vi "HFRR ADV v016 new software.vi"() -> ()   [LabVIEW 2025] (continued)
        n324 = event-data() -> ()  [unwired: 1 in, 6 out]
        n325 = Unbundle By Name("Password 3") -> ("Service Password"=w414:string)
        n326 = call <vilib>:"Trim Whitespace.vi"("string"=w414) -> ("trimmed string"=w412:string)  [unwired: 1 in]
        n327 = Equal?(x=w412, y="Service@123") -> (x = y?=w413:bool)
        n328 = case shown="False" w413 {
          selector: w413 -> [w418 w420]
          frame False {
            n329 = local write "Service Password enable"(w418) -> ()
            n330 = property on="Service Password Log" class="Str"("Visible"=TRUE) -> ()  [unwired: 2 in, 2 out]
            n331 = property on="Tab Control 5" class="TabCtl (strict)"("Tabs Visible?"=TRUE ("Page Labels Display Visible?")) -> ()  [unwired: 2 in, 2 out]
          }
          frame True {
            n332 = property on="Service Password Log" class="Str"("Visible"=FALSE) -> ()  [unwired: 2 in, 2 out]
            "Service Password enable" <- w420
          }
        }
      }
      event "Sign In": Value Change {
        w422 = FALSE ("Visible")
        n333 = event-data() -> ()  [unwired: 1 in, 6 out]
        n334 = property on="About" class="Clust (strict)"("Visible"=w422) -> ()  [unwired: 2 in, 2 out]
        n335 = property on="Password 3" class="Clust (strict)"("Visible"=w422) -> ()  [unwired: 2 in, 2 out]
        n336 = property on="Service Password Log" class="Str"("Visible"=FALSE) -> ()  [unwired: 2 in, 2 out]
      }
      event "Info": Value Change {
        n337 = event-data() -> ()  [unwired: 1 in, 6 out]
        n338 = local read "Info"() -> (w424:bool)
        n339 = case shown="False" w424 {
          frame False {
            n340 = property on="About" class="Clust (strict)"("Visible"=FALSE) -> ()  [unwired: 2 in, 2 out]
          }
          frame True {
            n341 = property on="About" class="Clust (strict)"("Visible"=TRUE) -> ()  [unwired: 2 in, 2 out]
          }
        }
      }
      event "Calibration": Value Change {
        n342 = event-data() -> ()  [unwired: 1 in, 6 out]
        n343 = local read "Calibration"() -> (w428:bool)
        n344 = case shown="False" w428 {
          frame False {
            n345 = property on="Calibration 2" class="TabCtl (strict)"("Visible"=FALSE) -> ()  [unwired: 2 in, 2 out]
            n346 = local write "Cal Password"("" ("Cal Password")) -> ()
          }
          frame True {
            n347 = property on="Calibration 2" class="TabCtl (strict)"("Visible"=TRUE) -> ()  [unwired: 2 in, 2 out]
            n348 = local write "Cal Password"("" ("Cal Password")) -> ()
          }
        }
        n349 = property on="Wrong Password" class="Str"("Visible"=FALSE) -> ()  [unwired: 2 in, 2 out]
      }
      event "Cal Password": Value Change {
        n350 = event-data() -> ()  [unwired: 1 in, 6 out]
        n351 = local read "Cal Password"() -> (w436:string)
        n352 = call <vilib>:"Trim Whitespace.vi"("string"=w436) -> ("trimmed string"=w435:string)  [unwired: 1 in]
        n353 = Equal?(x=w435, y="Cal@321") -> (x = y?=w433:bool)
        n354 = case shown="True" w433 {
          frame False {
            n355 = property on="Wrong Password" class="Str"("Visible"=TRUE) -> ()  [unwired: 2 in, 2 out]
          }
          frame True {
            n356 = property on="Wrong Password" class="Str"("Visible"=FALSE) -> ()  [unwired: 2 in, 2 out]
            n357 = local write "Main Tab"(T2."About" ("Main Tab")) -> ()
            n358 = local write "Cal Password"("" ("Cal Password")) -> ()
            n359 = local write "Main Dashboard Buttons"(T1."About" ("Main Dashboard Buttons")) -> ()
            n360 = local write "Tab Control 5"(T12."Temperature Calibration" ("Tab Control 5")) -> ()
            n361 = property on="Calibration 2" class="TabCtl (strict)"("Visible"=FALSE) -> ()  [unwired: 2 in, 2 out]
            n362 = property on="Tab Control 5" class="TabCtl (strict)"("Tabs Visible?"=FALSE ("Page Labels Display Visible?")) -> ()  [unwired: 2 in, 2 out]
            n363 = local write "Calibration"(FALSE ("Calibration")) -> ()
          }
        }
      }
      event "Calibration Selection": Value Change {
        n364 = event-data() -> ()  [unwired: 1 in, 6 out]
        n365 = local read "Calibration Selection"() -> (w447:T8)
        n366 = case shown="\"Stroke Calibration\"" w447 {
          tunnel: [T7."Stroke" ("Main Calibration Tab") T7."Friction" ("Main Calibration Tab") T7."Main" ("Main Calibration Tab") T7."Temperature" ("Main Calibration Tab")] -> w446
          frame "Stroke Calibration" {
          }
          frame "Friction Force Calibration" {
          }
          frame Default {
          }
          frame "Temperature Calibration" {
          }
        }
        n367 = local write "Main Calibration Tab"(w446) -> ()
      }
      event "Back Stroke": Value Change {
        n368 = event-data() -> ()  [unwired: 1 in, 6 out]
        n369 = local write "Main Stroke Tab"(T9."Step 1" ("Main Stroke Tab")) -> ()
        n370 = local write "Main Calibration Tab"(T7."Main" ("Main Calibration Tab")) -> ()
        n371 = local write "Back Stroke"(FALSE ("Back Stroke")) -> ()
      }
      event "Step 2 Back": Value Change {
        n372 = event-data() -> ()  [unwired: 1 in, 6 out]
        n373 = local write "Main Stroke Tab"(T9."Step 1" ("Main Stroke Tab")) -> ()
        n374 = local write "Step 2 Back"(FALSE ("Back Stroke")) -> ()
      }
      event "Step 3 Back": Value Change {
        n375 = event-data() -> ()  [unwired: 1 in, 6 out]
        n376 = local write "Main Stroke Tab"(T9."Step 2" ("Main Stroke Tab")) -> ()
        n377 = local write "Step 3 Back"(FALSE ("Back Stroke")) -> ()
      }
      event "Step 4 Back": Value Change {
        n378 = event-data() -> ()  [unwired: 1 in, 6 out]
        n379 = local write "Main Stroke Tab"(T9."Step 3" ("Main Stroke Tab")) -> ()
        n380 = local write "Step 4 Back"(FALSE ("Back Stroke")) -> ()
      }
      event "Step 5 Back": Value Change {
        n381 = event-data() -> ()  [unwired: 1 in, 6 out]
        n382 = local write "Main Stroke Tab"(T9."Step 4" ("Main Stroke Tab")) -> ()
        n383 = local write "Step 5 Back"(FALSE ("Back Stroke")) -> ()
      }
      event "Step 6 Back": Value Change {
        n384 = event-data() -> ()  [unwired: 1 in, 6 out]
        n385 = local write "Main Stroke Tab"(T9."Step 5" ("Main Stroke Tab")) -> ()
        n386 = local write "Step 6 Back"(FALSE ("Back Stroke")) -> ()
      }
      event "Back Stroke step 7": Value Change {
        n387 = event-data() -> ()  [unwired: 1 in, 6 out]
        n388 = local write "Main Stroke Tab"(T9."Step 6" ("Main Stroke Tab")) -> ()
        n389 = local write "Back Stroke step 7"(FALSE ("Back Stroke")) -> ()
      }
      event "Back Stroke step 8": Value Change {
        n390 = event-data() -> ()  [unwired: 1 in, 6 out]
        n391 = local write "Main Stroke Tab"(T9."Step 7" ("Main Stroke Tab")) -> ()
        n392 = local write "Back Stroke step 8"(FALSE ("Back Stroke")) -> ()
      }
      event "Back Stroke 8": Value Change {
        n393 = event-data() -> ()  [unwired: 1 in, 6 out]
        n394 = local write "MOVE CARRIAGE TO"(0.2 ("MOVE CARRIAGE TO")) -> ()
        n395 = local write "Main Stroke Tab"(T9."Step 1" ("Main Stroke Tab")) -> ()
        n396 = local write "Back Stroke 8"(FALSE ("Back Stroke 8")) -> ()
      }
      event "Continue Stroke": Value Change {
        n397 = event-data() -> ()  [unwired: 1 in, 6 out]
        n398 = local write "Main Stroke Tab"(T9."Step 2" ("Main Stroke Tab")) -> ()
        n399 = local write "Continue Stroke"(FALSE ("Continue Stroke")) -> ()
      }
      event "Continue Stroke step 2": Value Change {
        n400 = event-data() -> ()  [unwired: 1 in, 6 out]
        n401 = local write "Main Stroke Tab"(T9."Step 3" ("Main Stroke Tab")) -> ()
        n402 = local write "Continue Stroke step 2"(FALSE ("Continue Stroke")) -> ()
      }
      event "Continue Stroke step 3": Value Change {
        n403 = event-data() -> ()  [unwired: 1 in, 6 out]
        n404 = local write "Main Stroke Tab"(T9."Step 4" ("Main Stroke Tab")) -> ()
        n405 = local write "Continue Stroke step 3"(FALSE ("Continue Stroke")) -> ()
      }
      event "Continue Stroke step 4": Value Change {
        n406 = event-data() -> ()  [unwired: 1 in, 6 out]
        n407 = local write "Main Stroke Tab"(T9."Step 5" ("Main Stroke Tab")) -> ()
        n408 = local write "Continue Stroke step 4"(FALSE ("Continue Stroke")) -> ()
      }
      event "Continue Stroke step 5": Value Change {
        n409 = event-data() -> ()  [unwired: 1 in, 6 out]
        n410 = local write "Main Stroke Tab"(T9."Step 6" ("Main Stroke Tab")) -> ()
        n411 = local write "Continue Stroke step 5"(FALSE ("Continue Stroke")) -> ()
      }
      event "Continue Stroke step 6": Value Change {
        n412 = event-data() -> ()  [unwired: 1 in, 6 out]
        n413 = local write "Main Stroke Tab"(T9."Step 7" ("Main Stroke Tab")) -> ()
        n414 = local write "Continue Stroke step 6"(FALSE ("Continue Stroke")) -> ()
      }
      event "Continue Stroke step 7": Value Change {
        w486 = FALSE ("0.2mm")
        n415 = event-data() -> ()  [unwired: 1 in, 6 out]
        n416 = local write "0.4 mm"(w486) -> ()
        n417 = local write "0.6 mm"(w486) -> ()
        n418 = local write "1.0 mm"(w486) -> ()
        n419 = local write "1.2 mm"(w486) -> ()
        n420 = local write "0.2 2"(w486) -> ()
        n421 = local write "0.4 2"(w486) -> ()
        n422 = local write "0.6 2"(w486) -> ()
        n423 = local write "0.8 2"(w486) -> ()
        n424 = local write "1.0 2"(w486) -> ()
        n425 = local write "1.2"(w486) -> ()
        n426 = local write "0.2mm"(w486) -> ()
        n427 = local write "0.8mm"(w486) -> ()
        n428 = local write "Main Stroke Tab"(T9."Step 8" ("Main Stroke Tab")) -> ()
        n429 = local write "Continue Stroke step 7"(FALSE ("Continue Stroke")) -> ()
        n430 = local write "Stroke Test Complete"(T10."Test Progress" ("Stroke Test Complete")) -> ()
        "Position Measurment Temp" <- 0.0 ("Position Measurment Temp")
        "Calibration Tare" <- TRUE ("Calibration Tare")
        "MOVE CARRIAGE TO" <- 0.2 ("MOVE CARRIAGE TO")
      }
      event "Continue Stroke step 8": Value Change {
        n431 = event-data() -> ()  [unwired: 1 in, 6 out]
        n432 = local read "LVDT STROKE  Calibration"() -> (w491:dbl)
        n433 = local read "Position Measurment Temp"() -> (w492:dbl)
        n434 = case shown="4" w492 {
          selector: w492 -> [w497 w502 w507 w512 w517 w521 w524 w525]
          tunnel: w491 -> [w493 w498 w503 w508 w513 w518 _ _]
          frame 0, Default {
            w495 = TRUE ("0.2mm")
            n435 = Increment(x=w497) -> (x+1=w496:i32)
            n436 = local write "Position Measurment Temp"(w496) -> ()
            n437 = local write "0.2mm"(w495) -> ()
            n438 = local write "0.2 2"(w495) -> ()
            n439 = local write "MOVE CARRIAGE TO"(0.4 ("MOVE CARRIAGE TO")) -> ()
            "Calibration 0.2" <- w493
          }
          frame 1 {
            w500 = TRUE ("0.4 mm")
            n440 = Increment(x=w502) -> (x+1=w501:i32)
            n441 = local write "Calibration 0.4"(w498) -> ()
            n442 = local write "Position Measurment Temp"(w501) -> ()
            n443 = local write "0.4 mm"(w500) -> ()
            n444 = local write "MOVE CARRIAGE TO"(0.6 ("MOVE CARRIAGE TO")) -> ()
            n445 = local write "0.4 2"(w500) -> ()
          }
          frame 2 {
            w505 = TRUE ("0.6 mm")
            n446 = Increment(x=w507) -> (x+1=w506:i32)
            n447 = local write "Calibration 0.6"(w503) -> ()
            n448 = local write "Position Measurment Temp"(w506) -> ()
            n449 = local write "0.6 2"(w505) -> ()
            n450 = local write "0.6 mm"(w505) -> ()
            n451 = local write "MOVE CARRIAGE TO"(0.8 ("MOVE CARRIAGE TO")) -> ()
          }
          frame 3 {
            w509 = TRUE ("0.6 mm")
            n452 = Increment(x=w512) -> (x+1=w511:i32)
            n453 = local write "Position Measurment Temp"(w511) -> ()
            n454 = local write "MOVE CARRIAGE TO"(1.0 ("MOVE CARRIAGE TO")) -> ()
            n455 = local write "0.8mm"(w509) -> ()
            n456 = local write "0.8 2"(w509) -> ()
            "Calibration 0.8" <- w508
          }
          frame 4 {
            w514 = TRUE ("0.6 mm")
            n457 = Increment(x=w517) -> (x+1=w516:i32)
            n458 = local write "Position Measurment Temp"(w516) -> ()
            n459 = local write "MOVE CARRIAGE TO"(1.2 ("MOVE CARRIAGE TO")) -> ()
            n460 = local write "1.0 mm"(w514) -> ()
            n461 = local write "1.0 2"(w514) -> ()
            "Calibration 1.0" <- w513
          }
          frame 5 {
            w519 = TRUE ("0.6 mm")
            n462 = Increment(x=w521) -> (x+1=w520:i32)
            n463 = local write "Position Measurment Temp"(w520) -> ()
            n464 = local write "1.2 mm"(w519) -> ()
            n465 = local write "1.2"(w519) -> ()
            "Calibration 1.2" <- w518
          }
          frame 6 {
            n466 = Increment(x=w524) -> (x+1=w523:i32)
            n467 = local write "Position Measurment Temp"(w523) -> ()
            n468 = local write "Stroke Test Complete"(T10."Stroke Points Completed" ("Stroke Test Complete")) -> ()
          }
          frame 7 {
            n469 = stacked-sequence {
              tunnel: w525 -> [w526 _ _]
              frame #0 {
                n470 = Increment(x=w526) -> (x+1=w527:i32)
                n471 = local write "Main Stroke Tab"(T9."Step 9" ("Main Stroke Tab")) -> ()
                n472 = local write "Position Measurment Temp"(w527) -> ()
                n473 = Insert Into Array(array=dbl[] [], new element #1=0.2 ("new element/subarray"), new element #2=0.4 ("new element/subarray"), new element #3=0.6 ("new element/subarray"), new element #4=0.8 ("new element/subarray"), new element #5=1.0 ("new element/subarray"), new element #6=1.2 ("new element/subarray")) -> (→"1D stroke":dbl[])  [unwired: 1 in]
                n474 = local read "Calibration 0.2"() -> (w534:dbl)
                n475 = local read "Calibration 0.4"() -> (w533:dbl)
                n476 = local read "Calibration 0.6"() -> (w532:dbl)
                n477 = local read "Calibration 0.8"() -> (w531:dbl)
                n478 = local read "Calibration 1.0"() -> (w530:dbl)
                n479 = local read "Calibration 1.2"() -> (w529:dbl)
                n480 = Insert Into Array(array=dbl[] [], new element #1=w534, new element #2=w533, new element #3=w532, new element #4=w531, new element #5=w530, new element #6=w529) -> (→"Calibrated Voltage Value":dbl[])  [unwired: 1 in]
              }
              frame #1 {
                n481 = local read "Calibrated Voltage Value"() -> (w546:dbl[])
                n482 = local read "1D stroke"() -> (w547:dbl[])
                n483 = for {
                  tunnel: [w550] -> w545 mode=indexing
                  tunnel: w547 -> [w549] mode=indexing
                  tunnel: w546 -> [w548] mode=indexing
                  n484 = formula code="if (stroke == 0.2) {\n    status = (voltage >= 0.0961 && voltage <= 0.4961) ? 1 : 0;\n} else if (stroke == 0.4) {\n    status = (voltage >= 0.3425 && voltage <= 0.7425) ? 1 : 0;\n} else if (stroke == 0.6) {\n    status = (voltage >= 0.5370 && voltage <= 0.9370) ? 1 : 0;\n} else if (stroke == 0.8) {\n    status = (voltage >= 0.6640 && voltage <= 1.0640) ? 1 : 0;\n} else if (stroke == 1.0) {\n    status = (voltage >= 0.9000 && voltage <= 1.1000) ? 1 : 0;\n} else if (stroke == 1.2) {\n    status = (voltage >= 0.9278 && voltage <= 1.3278) ? 1 : 0;\n} else {\n    status = 0; // Fails if an invalid stroke value is supplied\n}"("stroke"=w549, "voltage"=w548) -> ("status"=w550:dbl)
                }
                "Status" <- w545
              }
              frame #2 {
                w557 = 1.0
                n485 = local read "Status"() -> (w564:dbl[])
                n486 = Index Array(array=w564) -> (element #1=w563:dbl, element #2=w562:dbl, element #3=w561:dbl, element #4=w560:dbl, element #5=w559:dbl, element #6=w558:dbl)  [unwired: 6 in]
                n487 = Equal?(x=w562, y=w557) -> (x = y?=w555:bool)
                n488 = Equal?(x=w561, y=w557) -> (x = y?=w554:bool)
                n489 = Equal?(x=w560, y=w557) -> (x = y?=w553:bool)
                n490 = Equal?(x=w559, y=w557) -> (x = y?=w552:bool)
                n491 = Equal?(x=w558, y=w557) -> (x = y?=w551:bool)
                n492 = Equal?(x=w563, y=w557) -> (x = y?=w556:bool)
                n493 = case shown="True" w556 {
                  selector: w556 -> [w575 w576]
                  frame True {
                    n494 = local write "Point 1 - 0.2 mm"(w575) -> ()
                    n495 = property on="Point 1 - 0.2 mm" class="Bool"("Caption.Visible"=w575) -> ()  [unwired: 2 in, 2 out]
                  }
                  frame False {
                    n496 = local write "Point 1 - 0.2 mm"(w576) -> ()
                    n497 = property on="Point 1 - 0.2 mm" class="Bool"("Caption.Visible"=w576) -> ()  [unwired: 2 in, 2 out]
                  }
                }
                n498 = case shown="True" w555 {
                  selector: w555 -> [w573 w574]
                  frame True {
                    n499 = local write "Point 2 - 0.4 mm"(w573) -> ()
                    n500 = property on="Point 2 - 0.4 mm" class="Bool"("Caption.Visible"=w573) -> ()  [unwired: 2 in, 2 out]
                  }
                  frame False {
                    n501 = local write "Point 2 - 0.4 mm"(w574) -> ()
                    n502 = property on="Point 2 - 0.4 mm" class="Bool"("Caption.Visible"=w574) -> ()  [unwired: 2 in, 2 out]
                  }
                }
                n503 = case shown="True" w552 {
                  selector: w552 -> [w567 w568]
                  frame True {
                    n504 = local write "Point 5 - 1.0 mm"(w567) -> ()
                    n505 = property on="Point 5 - 1.0 mm" class="Bool"("Caption.Visible"=w567) -> ()  [unwired: 2 in, 2 out]
                  }
                  frame False {
                    n506 = local write "Point 5 - 1.0 mm"(w568) -> ()
                    n507 = property on="Point 5 - 1.0 mm" class="Bool"("Caption.Visible"=w568) -> ()  [unwired: 2 in, 2 out]
                  }
                }
                n508 = case shown="True" w554 {
                  selector: w554 -> [w571 w572]
                  frame True {
                    n509 = local write "Point 3 - 0.6 mm"(w571) -> ()
                    n510 = property on="Point 3 - 0.6 mm" class="Bool"("Caption.Visible"=w571) -> ()  [unwired: 2 in, 2 out]
                  }
                  frame False {
                    n511 = local write "Point 3 - 0.6 mm"(w572) -> ()
                    n512 = property on="Point 3 - 0.6 mm" class="Bool"("Caption.Visible"=w572) -> ()  [unwired: 2 in, 2 out]
                  }
                }
                n513 = case shown="True" w553 {
                  selector: w553 -> [w569 w570]
                  frame True {
                    n514 = local write "Point 4 - 0.8 mm"(w569) -> ()
                    n515 = property on="Point 4 - 0.8 mm" class="Bool"("Caption.Visible"=w569) -> ()  [unwired: 2 in, 2 out]
                  }
                  frame False {
                    n516 = local write "Point 4 - 0.8 mm"(w570) -> ()
                    n517 = property on="Point 4 - 0.8 mm" class="Bool"("Caption.Visible"=w570) -> ()  [unwired: 2 in, 2 out]
                  }
                }
                n518 = case shown="True" w551 {
                  selector: w551 -> [w565 w566]
                  frame True {
                    n519 = local write "Point 6 - 1.2 mm"(w565) -> ()
                    n520 = property on="Point 6 - 1.2 mm" class="Bool"("Caption.Visible"=w565) -> ()  [unwired: 2 in, 2 out]
                  }
                  frame False {
                    n521 = local write "Point 6 - 1.2 mm"(w566) -> ()
                    n522 = property on="Point 6 - 1.2 mm" class="Bool"("Caption.Visible"=w566) -> ()  [unwired: 2 in, 2 out]
                  }
                }
              }
            }
          }
        }
      }
      event "TEMPERATURE STEP Back 1", "TEMPERATURE STEP Back air Temp": Value Change {
        n523 = event-data() -> ()  [unwired: 1 in, 6 out]
        n524 = stacked-sequence {
          frame #0 {
            n525 = local write "Main Calibration Tab"(T7."Main" ("Main Calibration Tab")) -> ()
          }
          frame #1 {
            n526 = Wait (ms)(milliseconds to wait=u32 1000) -> ()  [unwired: 1 out]
          }
          frame #2 {
            n527 = local write "Command"("CAL;END" ("Command")) -> ()
          }
          frame #3 {
            n528 = Wait (ms)(milliseconds to wait=u32 2000) -> ()  [unwired: 1 out]
          }
          frame #4 {
            n529 = local write "Command"("CAL;END" ("Command")) -> ()
          }
        }
      }
      event "Temperature Continue Step 1": Value Change {
        n530 = event-data() -> ()  [unwired: 1 in, 6 out]
        n531 = stacked-sequence {
          frame #0 {
            n532 = Wait (ms)(milliseconds to wait=u32 1500) -> ()  [unwired: 1 out]
          }
          frame #1 {
            n533 = local write "Command"("CAL;START" ("Command")) -> ()
          }
          frame #2 {
            n534 = Wait (ms)(milliseconds to wait=u32 1500) -> ()  [unwired: 1 out]
          }
          frame #3 {
            n535 = local write "Command"("CAL;START" ("Command")) -> ()
          }
          frame #4 {
            n536 = Wait (ms)(milliseconds to wait=u32 2000) -> ()  [unwired: 1 out]
          }
          frame #5 {
          }
          frame #6 {
            n537 = Wait (ms)(milliseconds to wait=u32 2000) -> ()  [unwired: 1 out]
          }
          frame #7 {
            # "CAL;A1;<true_T>"
            n538 = local write "Command"("CAL;A1;0" ("Command")) -> ()
          }
          frame #8 {
            n539 = local write "Tab Control 4"(T11."Step 2" ("Tab Control 4")) -> ()
          }
        }
      }
      event "Temperature Continue Step air Step 1": Value Change {
        n540 = event-data() -> ()  [unwired: 1 in, 6 out]
        n541 = stacked-sequence {
          frame #0 {
            n542 = Wait (ms)(milliseconds to wait=u32 1500) -> ()  [unwired: 1 out]
          }
          frame #1 {
            n543 = local write "Command"("CAL;START" ("Command")) -> ()
          }
          frame #2 {
            n544 = local write "Tab Control 4"(T11."Air Step 2" ("Tab Control 4")) -> ()
            n545 = Wait (ms)(milliseconds to wait=u32 1500) -> ()  [unwired: 1 out]
          }
          frame #3 {
            n546 = local write "Command"("CAL;START" ("Command")) -> ()
          }
          frame #4 {
            n547 = Wait (ms)(milliseconds to wait=u32 2000) -> ()  [unwired: 1 out]
          }
          frame #5 {
            # "CAL;A1;<true_T>"
            n548 = local write "Command"("CAL;A2;0" ("Command")) -> ()
          }
          frame #6 {
            n549 = Wait (ms)(milliseconds to wait=u32 2000) -> ()  [unwired: 1 out]
          }
          frame #7 {
            # "CAL;A1;<true_T>"
            n550 = local write "Command"("CAL;A1;0" ("Command")) -> ()
          }
        }
      }
      event "Temperature Selection": Value Change {
        n551 = event-data() -> ()  [unwired: 1 in, 6 out]
        n552 = local read "Temperature Selection"() -> (w599:enum32{"Air Temperature", "Sample Temperature"})
        n553 = case shown="\"Sample Temperature\"" w599 {
          frame "Air Temperature", Default {
            n554 = local write "Tab Control 4"(T11."Air Step 1" ("Tab Control 4")) -> ()
          }
          frame "Sample Temperature" {
            n555 = local write "Tab Control 4"(T11."Step 1" ("Tab Control 4")) -> ()
          }
        }
      }
      event "Temperature Continue Step 2": Value Change {
        n556 = event-data() -> ()  [unwired: 1 in, 6 out]
        n557 = stacked-sequence {
          frame #0 {
            n558 = stacked-sequence {
              frame #0 {
                n559 = Wait (ms)(milliseconds to wait=u32 1500) -> ()  [unwired: 1 out]
              }
              frame #1 {
                # "CAL;A1;<true_T>"
                n560 = local write "Command"("CAL;A1;0" ("Command")) -> ()
              }
              frame #2 {
                n561 = Wait (ms)(milliseconds to wait=u32 1500) -> ()  [unwired: 1 out]
              }
              frame #3 {
                # "CAL;A1;<true_T>"
                n562 = local write "Command"("CAL;A1;0" ("Command")) -> ()
              }
              frame #4 {
              }
            }
          }
          frame #1 {
            n563 = local write "Tab Control 4"(T11."Step 3" ("Tab Control 4")) -> ()
          }
        }
      }
      event "Temperature Continue Step 3": Value Change {
        n564 = event-data() -> ()  [unwired: 1 in, 6 out]
        n565 = stacked-sequence {
          frame #0 {
            n566 = stacked-sequence {
              frame #0 {
                n567 = Wait (ms)(milliseconds to wait=u32 1500) -> ()  [unwired: 1 out]
              }
              frame #1 {
              }
              frame #2 {
              }
              frame #3 {
                # "CAL;A1;<true_T>"
                n568 = local write "Command"("CAL;A1;60" ("Command")) -> ()
              }
              frame #4 {
                n569 = Wait (ms)(milliseconds to wait=u32 2000) -> ()  [unwired: 1 out]
              }
              frame #5 {
                # "CAL;A1;<true_T>"
                n570 = local write "Command"("CAL;A1;60" ("Command")) -> ()
              }
            }
          }
          frame #1 {
            n571 = Wait (ms)(milliseconds to wait=u32 1000) -> ()  [unwired: 1 out]
          }
          frame #2 {
            n572 = local write "Command"("CAL;SAVE" ("Command")) -> ()
          }
          frame #3 {
            n573 = Wait (ms)(milliseconds to wait=u32 1000) -> ()  [unwired: 1 out]
          }
          frame #4 {
            n574 = local write "Command"("CAL;SAVE" ("Command")) -> ()
          }
          frame #5 {
            n575 = Wait (ms)(milliseconds to wait=u32 1000) -> ()  [unwired: 1 out]
          }
          frame #6 {
            # "CAL;END"
            n576 = local write "Command"("CAL;END" ("Command")) -> ()
          }
          frame #7 {
            n577 = Wait (ms)(milliseconds to wait=u32 1000) -> ()  [unwired: 1 out]
          }
          frame #8 {
            # "CAL;END"
            n578 = local write "Command"("CAL;END" ("Command")) -> ()
          }
          frame #9 {
            n579 = local write "Main Calibration Tab"(T7."Temperature" ("Main Calibration Tab")) -> ()
            n580 = local write "Tab Control 4"(T11."Main" ("Tab Control 4")) -> ()
          }
        }
      }
      event "Back Stroke step main temperature": Value Change {
        n581 = event-data() -> ()  [unwired: 1 in, 6 out]
        n582 = stacked-sequence {
          frame #0 {
            n583 = Wait (ms)(milliseconds to wait=u32 1000) -> ()  [unwired: 1 out]
          }
          frame #1 {
            # "CAL;END"
            n584 = local write "Command"("CAL;END" ("Command")) -> ()
          }
          frame #2 {
            n585 = Wait (ms)(milliseconds to wait=u32 1000) -> ()  [unwired: 1 out]
          }
          frame #3 {
            # "CAL;END"
            n586 = local write "Command"("CAL;END" ("Command")) -> ()
          }
          frame #4 {
            n587 = local write "Main Calibration Tab"(T7."Temperature" ("Main Calibration Tab")) -> ()
            n588 = local write "Tab Control 4"(T11."Main" ("Tab Control 4")) -> ()
          }
        }
      }
      event "Quit": Value Change {
        n589 = event-data() -> ()  [unwired: 1 in, 6 out]
      }
    }
    n590 = Wait (ms)(milliseconds to wait=u32 100) -> ()  [unwired: 1 out]
  }
  n591 = while {
    stop <- w631 stop-if-true
    n592 = local read "Ambient Temperature"() -> (w629:dbl)
    n593 = local read "Sample Temperature"() -> (w628:dbl)
    n594 = local write "Temperature — Live (Set A: 60 °C)"(w628) -> ()
    n595 = local write "Temperature — Live (Set A: 60 °C)"(w628) -> ()
    n596 = local write "Temperature — Live (Set A: 0 °C)"(w629) -> ()
    n597 = local write "Sensor value"(w629) -> ()
    n598 = local write "Sensor value"(w628) -> ()
    n599 = local write "Temperature — Live (Set A: 60 °C)"(w629) -> ()
    n600 = local write "Sensor value"(w628) -> ()
    n601 = local write "Sensor value"(w629) -> ()
    n602 = Wait (ms)(milliseconds to wait=u32 200) -> ()  [unwired: 1 out]
    n603 = local read "Quit"() -> (w631:bool)
  }
  n604 = while {
    shift-right: [w633] -> _
    shift-left: "Enum - Selector" -> [w634]
    stop <- w635 stop-if-true
    # "Auto Start Logic Loop"
    n605 = case shown="\"Maintain Stage\"" w634 {
      tunnel: [w638 w644 w671 w703 w733 Auto_Start_enum."Exit" ("Enum - Selector") Auto_Start_enum."Init" ("Enum - Selector")] -> w633
      frame "Init", Default {
        n606 = local read "Auto Start Test"() -> (w637:bool)
        n607 = Select(t=Auto_Start_enum."Humidity & Temperature On" ("Enum - Selector"), s=w637, f=Auto_Start_enum."Init") -> (s? t:f=w638:T15)
      }
      frame "Humidity & Temperature On" {
        n608 = stacked-sequence {
          tunnel: [_ _ _ _ _ _ Auto_Start_enum."Reach point" ("Enum - Selector")] -> w641
          frame #0 {
            w646 = T18."Disabled and Grayed Out" ("Disabled")
            w647 = TRUE ("Heater Button")
            n609 = property on="Humidity" class="Bool (strict)"("DisabledEnum"=w646) -> ()  [unwired: 2 in, 2 out]
            n610 = property on="Heater Button" class="Bool (strict)"("DisabledEnum"=w646) -> ()  [unwired: 2 in, 2 out]
            n611 = local write "Heater Button"(w647) -> ()
            n612 = local write "Humidity"(w647) -> ()
            n613 = property on="Heater Button" class="Bool (strict)"("Val(Sgnl)"=TRUE ("Value (Signaling)")) -> ()  [unwired: 2 in, 2 out]
          }
          frame #1 {
            n614 = Wait (ms)(milliseconds to wait=u32 3000) -> ()  [unwired: 1 out]
          }
          frame #2 {
            n615 = local read "Set Temp"() -> (w653:dbl)
            n616 = Number To Fractional String(number=w653, precision (6)=i16 2) -> (F-format string=w650:string)  [unwired: 2 in]
            n617 = Concatenate Strings("ST;" ("Command"), w650) -> (w651:string)
            n618 = local write "Command"(w651) -> ()
          }
          frame #3 {
            n619 = Wait (ms)(milliseconds to wait=u32 1500) -> ()  [unwired: 1 out]
          }
          frame #4 {
            (unwired) i16 2 ("precision (6)")
            n620 = local read "Set Rh"() -> (w656:dbl)
            n621 = Number To Fractional String(number=w656) -> (F-format string=w659:string)  [unwired: 3 in]
            n622 = local read "WriteHumidity"() -> (w657:string[])
            n623 = Concatenate Strings("M;" ("new element/subarray"), w659) -> (w660:string)
            n624 = local write "Command"("HE;1" ("Command")) -> ()
            n625 = Insert Into Array(array=w657, new element=w660) -> (w658:string[])  [unwired: 1 in]
            n626 = local write "WriteHumidity"(w658) -> ()
          }
          frame #5 {
            n627 = Wait (ms)(milliseconds to wait=u32 1500) -> ()  [unwired: 1 out]
          }
          frame #6 {
            w663 = TRUE ("Reach point temp")
            n628 = local write "Reach point Humidity"(w663) -> ()
            n629 = local write "Reach point temp"(w663) -> ()
          }
        }
        n630 = local read "Auto Start Test"() -> (w643:bool)
        n631 = Not(x=w643) -> (.not. x?=w642:bool)
        n632 = Select(t=Auto_Start_enum."close", s=w642, f=w641) -> (s? t:f=w644:T15)
      }
      frame "Reach point" {
        w672 = TRUE ("PAUSE")
        w680 = 1.0 ("y")
        w683 = 1.0 ("y")
        n633 = local read "Set Temp"() -> (w665:dbl)
        n634 = local read "Set Humidity:"() -> (w679:dbl)
        n635 = local read "Humidity ( %RH )"() -> (w684:dbl)
        n636 = Add(x=w665, y=w683) -> (x+y=w682:dbl)
        n637 = Subtract(x=w665, y=w683) -> (x-y=w681:dbl)
        n638 = Add(x=w679, y=w680) -> (x+y=w678:dbl)
        n639 = Subtract(x=w679, y=w680) -> (x-y=w677:dbl)
        n640 = local read "TEMP"() -> (w685:dbl)
        n641 = In Range and Coerce(upper limit=w678, x=w684, lower limit=w677) -> (In Range?=w666:bool)  [unwired: 1 out]
        n642 = In Range and Coerce(upper limit=w682, x=w685, lower limit=w681) -> (In Range?=w667:bool)  [unwired: 1 out]
        n643 = case shown="True" w666 {
          frame False {
          }
          frame True {
            n644 = case shown="True" "Reach point Humidity" {
              selector: "Reach point Humidity" -> [_ w691]
              frame False {
              }
              frame True {
                n645 = local read "EVENT LOG"() -> (w688:string)
                n646 = Not(x=w691) -> (.not. x?=w690:bool)
                n647 = local write "Reach point Humidity"(w690) -> ()
                n648 = call "Event Log.vi"("Content"="Target Humidity reached", "EVENT LOG"=w688) -> ("EVENT LOG"=w689:string)  [unwired: 8 in, 1 out]
                n649 = local write "EVENT LOG"(w689) -> ()
              }
            }
          }
        }
        n650 = case shown="True" w667 {
          frame False {
          }
          frame True {
            n651 = case shown="True" "Reach point temp" {
              selector: "Reach point temp" -> [_ w697]
              frame False {
              }
              frame True {
                n652 = local read "EVENT LOG"() -> (w694:string)
                n653 = Not(x=w697) -> (.not. x?=w696:bool)
                n654 = local write "Reach point temp"(w696) -> ()
                n655 = call "Event Log.vi"("Content"="Target Temperature reached", "EVENT LOG"=w694) -> ("EVENT LOG"=w695:string)  [unwired: 8 in, 1 out]
                n656 = local write "EVENT LOG"(w695) -> ()
              }
            }
          }
        }
        n657 = local read "Auto Start Test"() -> (w670:bool)
        n658 = And(x=w667, y=w666) -> (x .and. y?=w676:bool)
        n659 = Select(t=Auto_Start_enum."Maintain Stage" ("Enum - Selector"), s=w676, f=Auto_Start_enum."Reach point" ("Enum - Selector")) -> (s? t:f=w673:T15)
        n660 = Not(x=w670) -> (.not. x?=w669:bool)
        n661 = Select(t=Auto_Start_enum."close", s=w669, f=w673) -> (s? t:f=w671:T15)
        n662 = call "ELAPSED TIMER VI.vi"("RESET"=w672, "PAUSE"=w672) -> ()  [unwired: 7 in, 3 out]
      }
      frame "Maintain Stage" {
        w712 = 2.0 ("y")
        w711 = 1.0 ("y")
        # "Humidity and  temperatures Set Point  have been reached"
        n663 = local read "Set Temp"() -> (w698:dbl)
        n664 = local read "Set Humidity:"() -> (w715:dbl)
        n665 = local read "Humidity ( %RH )"() -> (w718:dbl)
        n666 = Add(x=w698, y=w711) -> (x+y=w717:dbl)
        n667 = Subtract(x=w698, y=w711) -> (x-y=w716:dbl)
        n668 = local read "TEMP"() -> (w719:dbl)
        n669 = Add(x=w715, y=w712) -> (x+y=w714:dbl)
        n670 = Subtract(x=w715, y=w712) -> (x-y=w713:dbl)
        n671 = In Range and Coerce(upper limit=w717, x=w719, lower limit=w716) -> (In Range?=w710:bool)  [unwired: 1 out]
        n672 = In Range and Coerce(upper limit=w714, x=w718, lower limit=w713) -> (In Range?=w709:bool)  [unwired: 1 out]
        n673 = And(x=w710, y=w709) -> (x .and. y?=w708:bool)
        n674 = Not(x=w708) -> (.not. x?=w707:bool)
        n675 = call "ELAPSED TIMER VI.vi"("TARGET"=60.0, "RESET"=w707, "PAUSE"=FALSE) -> ("ELAPSED INDICATION"=w704:bool)  [unwired: 6 in, 2 out]
        n676 = case shown="True" w704 {
          tunnel: w704 -> [_ w722]
          tunnel: [Auto_Start_enum."Maintain Stage" ("Enum - Selector") w721] -> w702
          frame False {
          }
          frame True {
            n677 = stacked-sequence {
              tunnel: w722 -> [_ _ _ _ _]
              tunnel: [_ _ _ _ Auto_Start_enum."Start Stage" ("Enum - Selector")] -> w721
              frame #0 {
                n678 = local read "EVENT LOG"() -> (w724:string)
                n679 = call "Event Log.vi"("Content"="Humidity and temperature set point has stabilized.", "EVENT LOG"=w724) -> ("EVENT LOG"=w725:string)  [unwired: 8 in, 1 out]
                n680 = local write "EVENT LOG"(w725) -> ()
              }
              frame #1 {
                n681 = Wait (ms)(milliseconds to wait=u32 100) -> ()  [unwired: 1 out]
              }
              frame #2 {
                n682 = local read "EVENT LOG"() -> (w728:string)
                n683 = call "Event Log.vi"("Content"="Auto Test Started", "EVENT LOG"=w728) -> ("EVENT LOG"=w729:string)  [unwired: 8 in, 1 out]
                n684 = local write "EVENT LOG"(w729) -> ()
              }
              frame #3 {
                w730 = TRUE ("RUN")
                n685 = local write "RUN"(w730) -> ()
                n686 = property on="Auto Start Temp" class="Bool (strict)"("Val(Sgnl)"=w730) -> ()  [unwired: 2 in, 2 out]
                "Auto Start Temp" <- w730
              }
              frame #4 {
              }
            }
          }
        }
        n687 = local read "Auto Start Test"() -> (w701:bool)
        n688 = Not(x=w701) -> (.not. x?=w700:bool)
        n689 = Select(t=Auto_Start_enum."close", s=w700, f=w702) -> (s? t:f=w703:T15)
      }
      frame "Start Stage" {
        w732 = TRUE ("PAUSE")
        n690 = local read "Auto Start Test"() -> (w737:bool)
        n691 = Not(x=w737) -> (.not. x?=w736:bool)
        n692 = Select(t=Auto_Start_enum."close" ("Enum - Selector"), s=w736, f=Auto_Start_enum."Start Stage" ("Enum - Selector")) -> (s? t:f=w733:T15)
        n693 = call "ELAPSED TIMER VI.vi"("RESET"=w732, "PAUSE"=w732) -> ()  [unwired: 7 in, 3 out]
      }
      frame "close" {
        w739 = FALSE ("Heater Button")
        n694 = local write "RUN"(w739) -> ()
        n695 = local write "Heater Button"(w739) -> ()
        n696 = local write "Humidity"(w739) -> ()
        n697 = local write "Auto Start Test"(w739) -> ()
        n698 = property on="Heater Button" class="Bool (strict)"("Val(Sgnl)"=FALSE ("Value (Signaling)")) -> ()  [unwired: 2 in, 2 out]
      }
      frame "Exit" {
      }
    }
    n699 = Wait (ms)(milliseconds to wait=u32 100) -> ()  [unwired: 1 out]
    n700 = local read "Quit"() -> (w635:bool)
  }
  n701 = property on="Service Password Log" class="Str"("Visible"=w14) -> ()  [unwired: 2 in, 2 out]
  n702 = property on="Password 3" class="Clust (strict)"("Visible"=w14) -> ()  [unwired: 2 in, 2 out]
  n703 = while {
    stop <- w768 stop-if-true
    w751 = errorcluster {"status"=FALSE, "code"=0, "source"=""} ("error in (no error) 3")
    # "this loop is for manual report generation"
    n704 = local read "Confirm Measrurement"() -> (w750:bool)
    n705 = case shown="True" w750 {
      selector: w750 -> [_ w858]
      tunnel: errorcluster {"status"=FALSE, "code"=0, "source"=""} ("error in (no error) 3") -> [_ w859]
      tunnel: [_ w857] -> _
      frame False {
      }
      frame True {
        n706 = stacked-sequence {
          tunnel: w859 -> [_ w892 _]
          tunnel: w858 -> [_ _ w999]
          tunnel: [_ w880 _] -> w857
          frame #0 {
            n707 = String To Path(string="C:\\LAB-IQ\\Image Calibrate v01.dcf") -> (path=w862:path)
            n708 = Open/Create/Replace File ("Open File")(file path (use dialog)=w862) -> (refnum out=w863:refnum<file>)  [unwired: 5 in, 2 out]
            n709 = for {
              N: 4 -> [_]
              tunnel: w863 -> [w869]
              i -> [w865]
              n710 = Read from Text File ("Read File")(file (use dialog)=w869) -> (text=w870:string)  [unwired: 3 in, 3 out]
              n711 = String Subset(string=w870, offset (0)=6, length (rest)=10 ("length (rest)")) -> (substring=w866:string)
              n712 = Fract/Exp String To Number(string=w866) -> (number=w864:dbl)  [unwired: 3 in, 1 out]
              n713 = case shown="3" w865 {
                tunnel: w864 -> [w871 w872 _ w873 _]
                frame 0 {
                  n714 = local write "5x Gain"(w871) -> ()
                }
                frame 1 {
                  n715 = local write "10x Gain"(w872) -> ()
                }
                frame 2 {
                }
                frame 3 {
                  n716 = local write "100x gain"(w873) -> ()
                }
                frame 4, Default {
                }
              }
            }
          }
          frame #1 {
            n717 = local read "TEST STANDARD"() -> (w875:T3)
            n718 = case shown="\"ISO 12156\"" w875 {
              tunnel: ["ASTM D6079" "ISO 12156"] -> w874
              frame "ASTM D6079", Default {
              }
              frame "ISO 12156" {
              }
            }
            n719 = call "IMAGE ANALYSIS.vi"("Enum"=POST_ANALYSIS_ENUM."GET MEASUREMENTS", "error in"=w892) -> ("error out"=w899:errorcluster)  [unwired: 8 in, 1 out]
            n720 = local read "Magnification :"() -> (w885:string)
            n721 = call "Stall Data Flow.vim"("value in"=w899, "milliseconds to wait"=u32 1000) -> ("value out"=w898:errorcluster)  [unwired: 1 out]
            n722 = local read "Test File List :"() -> (w896:string)
            n723 = case shown="\"10x\"" w885 {
              tunnel: [w935 w936] -> w883
              frame "5x", Default {
                n724 = local read "5x Gain"() -> (w935:dbl)
              }
              frame "10x" {
                # "5x"
                n725 = local read "10x Gain"() -> (w936:dbl)
              }
            }
            n726 = call "IMAGE ANALYSIS.vi"("Enum"=POST_ANALYSIS_ENUM."READ", "error in"=w898) -> ("error out"=w895:errorcluster, "data out"=w886:string)  [unwired: 8 in]
            n727 = Match Pattern(string=w886, regular expression="\"type\": ") -> (after substring=w890:string)  [unwired: 1 in, 3 out]
            n728 = call "IMAGE PATH CREATION PY.vi"("error in (no error)"=w895, "File Name :"=w896) -> ("error out"=w894:errorcluster, "File Path"=w882:path, "File Path String:"=w877:string)  [unwired: 7 in]
            n729 = Match Pattern(string=w890, regular expression=",") -> (before substring=w876:string)  [unwired: 1 in, 3 out]
            n730 = local read "Calibration Tab"() -> (w879:enum32{"Measrument", "Calibrate"})
            n731 = call "Stall Data Flow.vim"("value in"=w894, "milliseconds to wait"=u32 250) -> ("value out"=w878:errorcluster)  [unwired: 1 out]
            n732 = Equal?(x=w876, y="\"rectangle\"") -> (x = y?=w887:bool)
            n733 = case shown="False" w887 {
              tunnel: w886 -> [w941 w996]
              tunnel: w883 -> [_ w987]
              tunnel: cluster{"major":dbl, "minor":dbl, "average":dbl} {"major"=0.0, "minor"=0.0, "average"=0.0} -> [w939 w983]
              tunnel: [w938 w980] -> w881
              tunnel: w876 -> [w940 _]
              tunnel: w883 -> [w937 _]
              frame False {
                n734 = Equal?(x=w940, y="\"line\"") -> (x = y?=w942:bool)
                n735 = case shown="True" w942 {
                  tunnel: w941 -> [_ w957]
                  tunnel: w939 -> [w944 w956]
                  tunnel: [w944 w954] -> w938
                  tunnel: w937 -> [_ w953]
                  frame False {
                  }
                  frame True {
                    w952 = 0.0 ("Major Axis")
                    n736 = Match Pattern(string=w957, regular expression="\"length_px\":") -> (after substring=w955:string)  [unwired: 1 in, 3 out]
                    n737 = property on="Major Axis" class="DigNum (strict)"("Caption.Text"="") -> ()  [unwired: 2 in, 2 out]
                    n738 = property on="Minor Axis" class="DigNum (strict)"("Caption.Text"="") -> ()  [unwired: 2 in, 2 out]
                    n739 = property on="Average" class="DigNum (strict)"("Caption.Text"="Line") -> ()  [unwired: 2 in, 2 out]
                    n740 = Fract/Exp String To Number(string=w955, default (0 dbl)=0.0 ("default (0 DBL)")) -> (number=w951:dbl)  [unwired: 2 in, 1 out]
                    "Pixel Value" <- w951
                    n741 = Multiply(x=w951, y=w953) -> (x*y=w964:dbl)
                    n742 = Multiply(x=w964, y=1000.0) -> (x*y=w947:dbl)
                    n743 = Divide(x=w947, y=1000.0) -> (x/y=w950:dbl)
                    n744 = local write "Measurment (mm)"(w950) -> ()
                    n745 = Bundle By Name(cluster=w956, "average"=w947) -> (w954:cluster{"major":dbl, "minor":dbl, "average":dbl})
                    n746 = Number To Fractional String(number=w947, precision (6)=i16 1) -> (F-format string=w946:string)  [unwired: 2 in]
                    n747 = local write "Minor Axis"(w952) -> ()
                    n748 = local write "Major Axis"(w952) -> ()
                    n749 = Fract/Exp String To Number(string=w946) -> (number=w945:dbl)  [unwired: 3 in, 1 out]
                    n750 = local write "Average"(w945) -> ()
                  }
                }
              }
              frame True {
                w984 = 1000.0 ("y")
                w990 = 0.0 ("default (0 DBL)")
                n751 = Match Pattern(string=w996, regular expression=" \"width_px\":") -> (after substring=w994:string)  [unwired: 1 in, 3 out]
                n752 = Match Pattern(string=w994, regular expression="\"height_px\":") -> (before substring=w992:string, after substring=w991:string)  [unwired: 1 in, 2 out]
                n753 = Fract/Exp String To Number(string=w992, default (0 dbl)=w990) -> (number=w989:dbl)  [unwired: 2 in, 1 out]
                n754 = Fract/Exp String To Number(string=w991, default (0 dbl)=w990) -> (number=w988:dbl)  [unwired: 2 in, 1 out]
                n755 = Multiply(x=w989, y=w987) -> (x*y=w986:dbl)
                n756 = Multiply(x=w988, y=w987) -> (x*y=w985:dbl)
                n757 = Multiply(x=w986, y=w984) -> (x*y=w970:dbl)
                n758 = Multiply(x=w985, y=w984) -> (x*y=w968:dbl)
                n759 = Add(x=w970, y=w968) -> (x+y=w982:dbl)
                n760 = property on="Major Axis" class="DigNum (strict)"("Caption.Text"="Major Axis") -> ()  [unwired: 2 in, 2 out]
                n761 = property on="Minor Axis" class="DigNum (strict)"("Caption.Text"="Minor Axis") -> ()  [unwired: 2 in, 2 out]
                n762 = property on="Average" class="DigNum (strict)"("Caption.Text"="Average") -> ()  [unwired: 2 in, 2 out]
                n763 = Divide(x=w982, y=2.0) -> (x/y=w966:dbl)
                n764 = Bundle By Name(cluster=w983, "major"=w970, "minor"=w968, "average"=w966) -> (w980:cluster{"major":dbl, "minor":dbl, "average":dbl})
                n765 = Number To Fractional String(number=w968, precision (6)=i16 1) -> (F-format string=w975:string)  [unwired: 2 in]
                n766 = Number To Fractional String(number=w966, precision (6)=i16 1) -> (F-format string=w976:string)  [unwired: 2 in]
                n767 = Number To Fractional String(number=w970, precision (6)=i16 1) -> (F-format string=w974:string)  [unwired: 2 in]
                n768 = Fract/Exp String To Number(string=w975) -> (number=w967:dbl)  [unwired: 3 in, 1 out]
                n769 = Fract/Exp String To Number(string=w976) -> (number=w965:dbl)  [unwired: 3 in, 1 out]
                n770 = Fract/Exp String To Number(string=w974) -> (number=w969:dbl)  [unwired: 3 in, 1 out]
                n771 = local write "Major Axis"(w969) -> ()
                n772 = local write "Average"(w965) -> ()
                n773 = local write "Minor Axis"(w967) -> ()
              }
            }
            n774 = case shown="\"Measrument\", Default" w879 {
              tunnel: w882 -> [w909 _]
              tunnel: w881 -> [w908 _]
              tunnel: [w905 w934] -> w880
              tunnel: w878 -> [w907 w934]
              tunnel: w877 -> [w906 _]
              tunnel: w874 -> [w904 _]
              frame "Measrument", Default {
                n775 = stacked-sequence {
                  tunnel: w909 -> [w927 _]
                  tunnel: w908 -> [w925 _]
                  tunnel: w907 -> [w923 _]
                  tunnel: w906 -> [w922 _]
                  tunnel: [w917 _] -> w905
                  tunnel: w904 -> [w910 _]
                  frame #0 {
                    n776 = call "IMAGE ANALYSIS.vi"("Enum"=POST_ANALYSIS_ENUM."SAVE IMAGE", "error in"=w923, "IMAGE FILE PATH"=w922) -> ("error out"=w921:errorcluster)  [unwired: 7 in, 1 out]
                    n777 = call "Stall Data Flow.vim"("value in"=w921, "milliseconds to wait"=u32 1000) -> ("value out"=w912:errorcluster)  [unwired: 1 out]
                    n778 = local read "Test File List :"() -> (w929:string)
                    n779 = call "IMAGE ANALYSIS.vi"("Enum"=POST_ANALYSIS_ENUM."MINIMIZE UI", "error in"=w912) -> ("error out"=w919:errorcluster)  [unwired: 8 in, 1 out]
                    n780 = Bundle By Name(cluster=T25 {"File Name"="", "Test Method"="", "Operator"="", "Fuel Description"="", "Date and time"=""} ("Main Ref"), "Test Method"=w910, "File Name"=w929) -> (w930:T25)
                    n781 = call "Stall Data Flow.vim"("value in"=w919, "milliseconds to wait"=u32 1500) -> ("value out"=w914:errorcluster)  [unwired: 1 out]
                    n782 = call "duf file read.vi"("error in (no error)"=w914, "Main Ref"=w930) -> ("error out"=w928:errorcluster, "Main Ref 2"=w926:T25)  [unwired: 8 in]
                    n783 = call "DETECTION REPORT for manual.vi"("error in (no error)"=w928, "return value 3"=w925, "Image File Path"=w927, "Main Ref"=w926) -> ("error out"=w924:errorcluster)  [unwired: 7 in]
                    n784 = call <vilib>:"Clear Errors.vi"("error in (no error)"=w924) -> ("error out"=w915:errorcluster)  [unwired: 5 in, 1 out]
                    n785 = call "IMAGE ANALYSIS.vi"("Enum"=POST_ANALYSIS_ENUM."MINIMIZE UI", "error in"=w915) -> ("error out"=w917:errorcluster)  [unwired: 8 in, 1 out]
                  }
                  frame #1 {
                    n786 = local write "Main Tab"(T2."HOME" ("Main Tab")) -> ()
                    n787 = local write "Main Dashboard Buttons"(T1."Home" ("Main Dashboard Buttons")) -> ()
                  }
                }
              }
              frame "Calibrate" {
              }
            }
          }
          frame #2 {
            n788 = Not(x=w999) -> (.not. x?=w998:bool)
            n789 = local write "Confirm Measrurement"(w998) -> ()
            n790 = local read "Calibration Tab"() -> (w997:enum32{"Measrument", "Calibrate"})
            n791 = case shown="\"Measrument\", Default" w997 {
              frame "Measrument", Default {
                (unwired) T20."HOME" ("Main Tab")
                n792 = local write "Main Tab"(T2."HOME" ("Main Tab")) -> ()
              }
              frame "Calibrate" {
              }
            }
          }
        }
      }
    }
    n793 = local read "Humidity"() -> (w742:bool)
    n794 = local read "Save Change"() -> (w747:bool)
    n795 = local read "Calibrate"() -> (w748:bool)
    n796 = local read "Auto Start Test"() -> (w743:bool)
    n797 = case shown="True" w748 {
      selector: w748 -> [_ w855]
      frame False {
      }
      frame True {
        n798 = Not(x=w855) -> (.not. x?=w854:bool)
        n799 = local write "Calibrate"(w854) -> ()
        n800 = local write "Calibration Tab"(enum32{"Measrument", "Calibrate"}."Calibrate" ("Calibration Tab")) -> ()
      }
    }
    n801 = case shown="True" w747 {
      selector: w747 -> [_ w799]
      frame False {
      }
      frame True {
        n802 = stacked-sequence {
          tunnel: w799 -> [_ _ _ _ w853]
          frame #0 {
            n803 = call "IMAGE ANALYSIS.vi"("Enum"=POST_ANALYSIS_ENUM."HIDE UI") -> ()  [unwired: 9 in, 2 out]
          }
          frame #1 {
            n804 = local read "100x gain"() -> (w801:dbl)
            n805 = local read "10x Gain"() -> (w802:dbl)
            n806 = local read "5x Gain"() -> (w803:dbl)
            n807 = Number To Fractional String(number=w802, width (-)=i16 4, precision (6)=i16 7) -> (F-format string=w824:string)  [unwired: 1 in]
            n808 = Number To Fractional String(number=0.0, width (-)=i16 4, precision (6)=i16 7) -> (F-format string=w819:string)  [unwired: 1 in]
            n809 = Number To Fractional String(number=w801, width (-)=i16 4, precision (6)=i16 7) -> (F-format string=w807:string)  [unwired: 1 in]
            n810 = Number To Fractional String(number=w803, width (-)=i16 10 ("precision (6)"), precision (6)=i16 7) -> (F-format string=w833:string)  [unwired: 1 in]
            n811 = Concatenate Strings("[CH1]" ("string"), w833, " - 5x Gain" ("string"), "\r") -> (w823:string)
            n812 = Concatenate Strings("[CH2]" ("string"), w824, " - 10x Gain" ("string"), "\r") -> (w822:string)
            n813 = Concatenate Strings("[CH3]" ("string"), w819, " - 20x Gain" ("string"), "\r") -> (w813:string)
            n814 = Concatenate Strings("[CH4]" ("string"), w807, " - 100x Gain" ("string"), "\r") -> (w806:string)
            n815 = String To Path(string="C:\\LAB-IQ\\Image Calibrate v01.dcf") -> (path=w836:path)
            n816 = Concatenate Strings(w823, w822, w813, w806) -> (w821:string)
            n817 = call <vilib>:"Write Characters To File.vi"("append to file? (new file:F)"=FALSE, "character string"=w821, "file path (dialog if empty)"=w836) -> ()  [unwired: 2 in, 1 out]
          }
          frame #2 {
            n818 = String To Path(string="C:\\LAB-IQ\\Image Calibrate v01.dcf") -> (path=w839:path)
            n819 = Open/Create/Replace File ("Open File")(file path (use dialog)=w839) -> (refnum out=w840:refnum<file>)  [unwired: 5 in, 2 out]
            n820 = for {
              N: 4 -> [_]
              tunnel: w840 -> [w846]
              i -> [w842]
              n821 = Read from Text File ("Read File")(file (use dialog)=w846) -> (text=w847:string)  [unwired: 3 in, 3 out]
              n822 = String Subset(string=w847, offset (0)=6, length (rest)=10 ("length (rest)")) -> (substring=w843:string)
              n823 = Fract/Exp String To Number(string=w843) -> (number=w841:dbl)  [unwired: 3 in, 1 out]
              n824 = case shown="3" w842 {
                tunnel: w841 -> [w848 w849 _ w850 _]
                frame 0 {
                  n825 = local write "5x Gain"(w848) -> ()
                }
                frame 1 {
                  n826 = local write "10x Gain"(w849) -> ()
                }
                frame 2 {
                }
                frame 3 {
                  n827 = local write "100x gain"(w850) -> ()
                }
                frame 4, Default {
                }
              }
            }
          }
          frame #3 {
            n828 = call "IMAGE ANALYSIS.vi"("Enum"=POST_ANALYSIS_ENUM."SHOW UI") -> ()  [unwired: 9 in, 2 out]
          }
          frame #4 {
            n829 = Not(x=w853) -> (.not. x?=w852:bool)
            n830 = local write "Save Change"(w852) -> ()
          }
        }
      }
    }
    n831 = case shown="False" w743 {
      tunnel: w742 -> [w769 _]
      frame False {
        n832 = case shown="True" w769 {
          frame False {
          }
          frame True {
            n833 = local read "Set Humidity:"() -> (w773:dbl)
            n834 = local read "Set Humidity:"() -> (w776:dbl)
            n835 = local read "Humidity ( %RH )"() -> (w777:dbl)
            n836 = Subtract(x=w773, y=2.0) -> (x-y=w771:dbl)
            n837 = Add(x=w776, y=2.0) -> (x+y=w772:dbl)
            n838 = In Range and Coerce(upper limit=w772, x=w777, lower limit=w771) -> (In Range?=w770:bool)  [unwired: 1 out]
            n839 = case shown="True" w770 {
              frame False {
              }
              frame True {
                n840 = case shown="True" "Manual Humididty Reached" {
                  selector: "Manual Humididty Reached" -> [_ w780]
                  frame False {
                  }
                  frame True {
                    n841 = Not(x=w780) -> (.not. x?=w779:bool)
                    n842 = local write "Manual Humididty Reached"(w779) -> ()
                    n843 = local read "EVENT LOG"() -> (w782:string)
                    n844 = call "Event Log.vi"("Content"="Target Humidity reached", "EVENT LOG"=w782) -> ("EVENT LOG"=w781:string)  [unwired: 8 in, 1 out]
                    n845 = local write "EVENT LOG"(w781) -> ()
                  }
                }
              }
            }
          }
        }
      }
      frame True {
        n846 = local write "Manual Humididty Reached"(TRUE ("Manual Humididty Reached")) -> ()
      }
    }
    n847 = local read "Cap Live Image"() -> (w763:bool)
    n848 = local read "SCAR MEASURMENT"() -> (w766:enum32{"Auto Scar", "Manual Scar"})
    n849 = Wait (ms)(milliseconds to wait=u32 250) -> ()  [unwired: 1 out]
    n850 = Equal?(x=w766, y=enum32{"Auto Scar", "Manual Scar"}."Manual Scar" ("SCAR MEASURMENT")) -> (x = y?=w764:bool)
    n851 = And(x=w764, y=w763) -> (x .and. y?=w762:bool)
    n852 = case shown="True" w762 {
      selector: w762 -> [_ w1078]
      frame False {
      }
      frame True {
        n853 = stacked-sequence {
          tunnel: [_ _ _ w1093 _] -> _
          tunnel: w1078 -> [_ _ _ _ w1100]
          frame #0 {
            w1079 = 0.0
            n854 = local write "Major Axis"(w1079) -> ()
            n855 = local write "Minor Axis"(w1079) -> ()
            n856 = local write "Average"(w1079) -> ()
          }
          frame #1 {
            n857 = call "CAMERA LIVE FEED FGV.vi"("Enum - Menu"=CAMERA_LIVE_FEED_ENUM."CAMERA MINIMIZE") -> ()  [unwired: 9 in, 2 out]
          }
          frame #2 {
            n858 = local read "FILE 3"() -> (w1087:string)
            n859 = call <vilib>:"Trim Whitespace.vi"("string"="C:\\LAB-IQ\\images\\") -> ("trimmed string"=w1089:string)  [unwired: 1 in]
            n860 = String To Path(string=w1089) -> (path=w1088:path)
            n861 = Concatenate Strings(w1087, ".png" ("string")) -> (w1086:string)
            n862 = Build Path(base path=w1088, name or relative path=w1086) -> (appended path=w1084:path)
            n863 = Path To String(path=w1084) -> (string=w1083:string)
            n864 = call "CAMERA LIVE FEED FGV.vi"("Enum - Menu"=CAMERA_LIVE_FEED_ENUM."CAMERA SAVE", "Image Path"=w1083) -> ("error out"=w1081:errorcluster)  [unwired: 8 in, 1 out]
            n865 = case shown="No Error" w1081 {
              frame No Error {
                n866 = One Button Dialog(message="Image saved successfully") -> ()  [unwired: 1 in, 1 out]
              }
              frame Error {
              }
            }
          }
          frame #3 {
            n867 = call "LIST FILE NAMES.vi"() -> ("error out"=w1095:errorcluster, "filenames"=w1092:string[])  [unwired: 10 in]
            n868 = call "IMAGE ANALYSIS.vi"("Enum"=POST_ANALYSIS_ENUM."SHOW UI", "error in"=w1095) -> ("error out"=w1093:errorcluster)  [unwired: 8 in, 1 out]
            n869 = property on="Test File List :" class="CmbBox"("Strings[]"=w1092) -> ()  [unwired: 2 in, 2 out]
          }
          frame #4 {
            (unwired) T24."Report" ("Main Dashboard Buttons")
            (unwired) T26."Report" ("Main Dashboard Buttons")
            n870 = Not(x=w1100) -> (.not. x?=w1099:bool)
            n871 = local write "Zoom Factore"(0.0 ("Zoom Factore")) -> ()
            n872 = local write "Cap Live Image"(w1099) -> ()
            n873 = local write "Main Tab"(T2."Adv Scar Report" ("Main Tab")) -> ()
            n874 = property on="Cap Live Image" class="Bool (strict)"("BoolText.Text"="Capture Image" ("Boolean Text.Text")) -> ()  [unwired: 2 in, 2 out]
            n875 = local write "Main Dashboard Buttons"(T1."Report" ("Main Dashboard Buttons")) -> ()
          }
        }
      }
    }
    n876 = local read "change Gain"() -> (w746:bool)
    n877 = local read "Back Square"() -> (w745:bool)
    n878 = case shown="True" w746 {
      selector: w746 -> [_ w790]
      frame False {
      }
      frame True {
        n879 = stacked-sequence {
          tunnel: w790 -> [_ w798]
          frame #0 {
            n880 = local read "Actual (µm)"() -> (w794:dbl)
            n881 = local read "Pixel Value"() -> (w793:dbl)
            n882 = local read "Magnification :"() -> (w792:string)
            n883 = Divide(x=w794, y=w793) -> (x/y=w791:dbl)
            n884 = case shown="\"10x\"" w792 {
              tunnel: w791 -> [w795 w796]
              frame "10x" {
                n885 = local write "10x Gain"(w795) -> ()
              }
              frame "5x", Default {
                n886 = local write "5x Gain"(w796) -> ()
              }
            }
          }
          frame #1 {
            n887 = Not(x=w798) -> (.not. x?=w797:bool)
            n888 = local write "change Gain"(w797) -> ()
          }
        }
      }
    }
    n889 = case shown="True" w745 {
      selector: w745 -> [_ w788]
      frame False {
      }
      frame True {
        n890 = Not(x=w788) -> (.not. x?=w787:bool)
        n891 = local write "Back Square"(w787) -> ()
        n892 = local write "Calibration Tab"(enum32{"Measrument", "Calibrate"}."Measrument" ("Calibration Tab")) -> ()
      }
    }
    n893 = local read "Rectangle Tool"() -> (w757:bool)
    n894 = local read "Clear ROI Tool"() -> (w756:bool)
    n895 = local read "Open Image"() -> (w761:bool)
    n896 = local read "line tool"() -> (w758:bool)
    n897 = local read "OUT"() -> (w759:bool)
    n898 = local read "In"() -> (w760:bool)
    n899 = case shown="True" w761 {
      selector: w761 -> [_ w1066]
      tunnel: [w1062 w1068] -> _
      tunnel: w751 -> [w1062 w1067]
      frame False {
      }
      frame True {
        n900 = Not(x=w1066) -> (.not. x?=w1065:bool)
        n901 = local write "Open Image"(w1065) -> ()
        n902 = call "IMAGE ANALYSIS.vi"("Enum"=POST_ANALYSIS_ENUM."HIDE UI", "error in"=w1067) -> ("error out"=w1075:errorcluster)  [unwired: 8 in, 1 out]
        n903 = call "File Dialog"("start path"=path "C:/LAB-IQ/images", "error in"=w1075) -> ("selected path"=w1064:path, "error out"=w1073:errorcluster)  [unwired: 10 in, 2 out]
        "Image path  2" <- w1064
        n904 = call <vilib>:"Clear Errors.vi"("error in (no error)"=w1073) -> ("error out"=w1072:errorcluster)  [unwired: 5 in, 1 out]
        n905 = call "IMAGE ANALYSIS.vi"("Enum"=POST_ANALYSIS_ENUM."OPEN FILE", "error in"=w1072, "File Path"=w1064) -> ("error out"=w1071:errorcluster)  [unwired: 7 in, 1 out]
        n906 = call <vilib>:"Clear Errors.vi"("error in (no error)"=w1071) -> ("error out"=w1070:errorcluster)  [unwired: 5 in, 1 out]
